vi "Manual Intake Mode.vi"(6 "Current Encoder Position":dbl) -> (1 "Rollers Active?":bool, 2 "Arm Power":dbl, 3 "Intake Power":dbl)   [LabVIEW 2015]
uses:
  Robot Global Data.vi
  <vilib>/addons/control/pid/pid.llb/PID (DBL).vi
  <vilib>/addons/control/pid/NI_PID_pid.lvlib
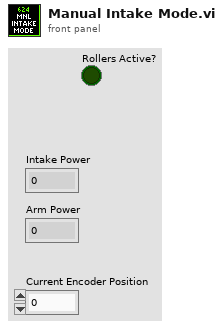
[diagram p1: front panel]
types:
  T1 = typedef "Dashboard Control Data.ctl" = cluster{"Encoder Control":T2, "Steer PID output":cluster{"output high":dbl, "output low":dbl}, " Steer PID gains":cluster{"proportional gain (Kc)":dbl, "integral time (Ti, min)":dbl, "derivative time (Td, min)":dbl}, "Drivetrain Settings":T3, "Vision Packet":T4, "Dashboard Drivetrain Command":T5, "Info/Command Cluster":T7, "Ball Vision Packet":T8, "Intake Presets":T10, "Intake Encoder Control":T12, "Climb Presets":T13, "Goal Output Range":cluster{"output high":dbl, "output low":dbl}, "Enabled Systems":T14, "Auton Presets":T15, "Pressure M":dbl, "Pressure B":dbl, "Vision Timeout":dbl, "Auto-Shift":T16, "Catapult Setpoints":T17}
  T2 = typedef "Encoder Control.ctl" = cluster{"Right Tick Constant":dbl, "Left Tick Constant":dbl, "Reset?":bool, "Y Dist":cluster{"PID gains":cluster{"proportional gain (Kc)":dbl, "integral time (Ti, min)":dbl, "derivative time (Td, min)":dbl}}, "Y Stop Thresh":dbl, "Y Stop Speed":dbl}
  T3 = typedef "Drivetrain Settings.ctl" = cluster{"Gyro Tolerance":dbl, "Throttle Ramp (ms)":dbl, "Kv":dbl, "Ka":dbl, "Feed Forward P":dbl, "Feed Forward D":dbl, "Goal Vision PID gains":cluster{"proportional gain (Kc)":dbl, "integral time (Ti, min)":dbl, "derivative time (Td, min)":dbl}, "Goal Detection Window":dbl, "Creep Rate":dbl, "Vision Throttle Threshold":dbl, "Min Turn Output":dbl, "Left Batter Angle":dbl, "Right Batter Angle":dbl}
  T4 = typedef "Goal Vision Packet.ctl" = cluster{"Distance":dbl, "Center X":dbl, "Center Y":dbl, "Found Target?":bool, "Robot Center":dbl, "Angle":dbl}
  T5 = typedef "Dashboard Drivetrain Command.ctl" = cluster{"Drivetrain Vision":T6}
  T6 = typedef "Drivetrain Vision.ctl" = cluster{"Goal Window":dbl, "Ball Window":dbl}
  T7 = typedef "Ball Tracking Command Cluster.ctl" = cluster{"Distance to Ball":dbl, "Desired Angle":dbl, "Command":enum16{"Turn to Ball", "Turn to Angle", "Get Distance"}, "Pixels from Center":dbl}
  T8 = typedef "Ball Vision Packet.ctl" = cluster{"Ball Detected?":bool, "Distance to Ball":dbl, "Desired Angle":dbl, "Pixels from Center":dbl, "Tracking mode":T9}
  T9 = typedef "Tracking Mode.ctl" = enum16{"Turn to Ball", "Turn to Angle"}
  T10 = typedef "Intake Presets.ctl" = cluster{"Intake Speed":dbl, "Outake Speed":dbl, "Angle Speed":dbl, "Angle Tolerance":dbl, "Encoder Scale":dbl, "Load Height":dbl, "Output Range":T11, "MaxCurrent":dbl, "Idle Height":dbl, "Max Height":dbl, "Reset Encoders?":bool, "PID gains":cluster{"proportional gain (Kc)":dbl, "integral time (Ti, min)":dbl, "derivative time (Td, min)":dbl}, "Drop Low Height ":dbl, "Rotation Power Max/Min":dbl}
  T11 = typedef "Drivetrain Output Range.ctl" = cluster{"output high":dbl, "output low":dbl}
  T12 = typedef "IntakeEcoderControl.ctl" = cluster{"Arm Tick Constant":dbl, "Reset?":bool, "Y Dist":cluster{"PID gains":cluster{"proportional gain (Kc)":dbl, "integral time (Ti, min)":dbl, "derivative time (Td, min)":dbl}}, "Y Stop Thresh":dbl, "Y Stop Speed":dbl}
  T13 = typedef "Climb Presets.ctl" = cluster{"Pull Power":dbl, "Extend Power":dbl}
  T14 = typedef "Enabled Systems.ctl" = cluster{"Shoot":bool, "Intake":bool, "DT":bool, "Gyro":bool, "100ms":bool, "US":bool}
  T15 = typedef "Autonomous Presets.ctl" = cluster{"Pitch Limit":dbl, "Roll Limit":dbl, "Start Position":dbl, "Cross Position":dbl}
  T16 = typedef "Auto Shift Cluster.ctl" = cluster{"Delay":dbl, "Speed Thresh":dbl, "Upshift Accel":dbl, "Upshift Throttle":dbl, "Upshift Throttle Accel":dbl, "Downshift Throttle":dbl, "Downshift Throttle Accel":dbl, "Pressure Threshold":dbl}
  T17 = typedef "Catapult Presets.ctl" = cluster{"Intake Danger Height":dbl, "Ball Security Delay ":dbl, "High PSI Minimum":dbl, "Shot Finish Delay":dbl, "Low PSI Minimum":dbl, "Idle Ball Security Wait ":dbl}
  T18 = typedef "Manual Intake Commands.ctl" = cluster{"Intake":bool, "Eject":bool, "Arm Angle":dbl, "Intake Override Speed":dbl, "Arm Override Speed":dbl, "Arm Speed":dbl, "Override Intake":bool, "Override Eject":bool, "Eject Override Speed":dbl, "Arm":bool, "Override Arm":bool, "Override Angle":bool}
  T19 = cluster{"proportional gain (Kc)":dbl, "integral time (Ti, min)":dbl, "derivative time (Td, min)":dbl}
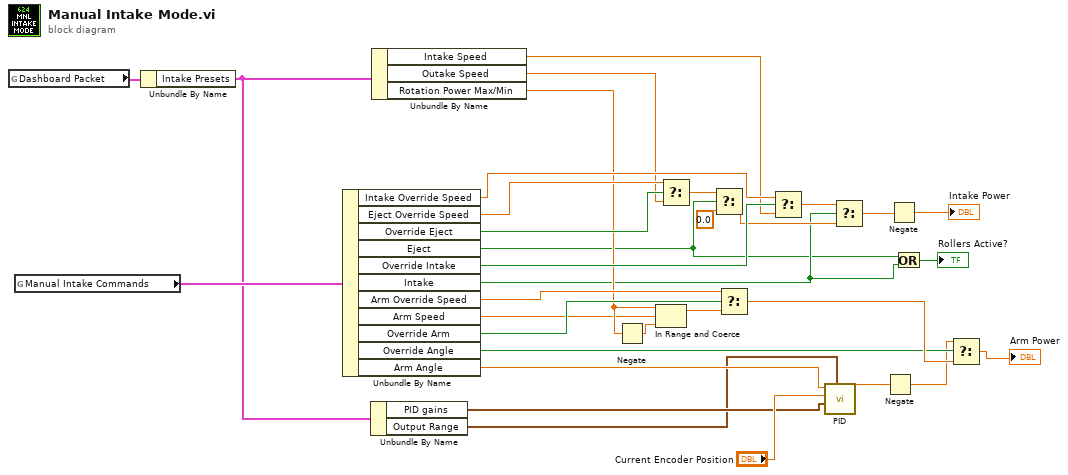
[diagram p0: block diagram]
diagram:
  n1 = global read "Robot Global Data.vi" "Dashboard Packet"() -> (w24:T1)
  n2 = global read "Robot Global Data.vi" "Manual Intake Commands"() -> (w21:T18)
  n3 = Unbundle By Name(w24) -> ("Intake Presets"=w8:T10)
  n4 = Unbundle By Name(w21) -> ("Intake Override Speed"=w27:dbl, "Eject Override Speed"=w33:dbl, "Override Eject"=w32:bool, "Eject"=w12:bool, "Override Intake"=w29:bool, "Intake"=w13:bool, "Arm Override Speed"=w25:dbl, "Arm Speed"=w17:dbl, "Override Arm"=w20:bool, "Override Angle"=w4:bool, "Arm Angle"=w10:dbl)
  n5 = Unbundle By Name(w8) -> ("PID gains"=w7:T19, "Output Range"=w6:T11)
  n6 = Unbundle By Name(w8) -> ("Intake Speed"=w23:dbl, "Outake Speed"=w22:dbl, "Rotation Power Max/Min"=w19:dbl)
  n7 = Negate(x=w19) -> (-x=w18:dbl)
  n8 = In Range and Coerce(upper limit=w19, x=w17, lower limit=w18) -> (coerced(x)=w16:dbl)  [unwired: 1 out]
  n9 = Select(t=w33, s=w32, f=w22) -> (s? t:f=w31:dbl)
  n10 = Select(t=w31, s=w12, f=0.0) -> (s? t:f=w26:dbl)
  n11 = Select(t=w25, s=w20, f=w16) -> (s? t:f=w5:dbl)
  n12 = Select(t=w27, s=w29, f=w23) -> (s? t:f=w30:dbl)
  n13 = call-poly <vilib>:"PID.vi"("output range"=w6, "PID gains"=w7, "process variable"="Current Encoder Position", "setpoint"=w10) -> ("output"=w3:dbl)  [unwired: 6 in, 1 out]
  n14 = Select(t=w30, s=w13, f=w26) -> (s? t:f=w15:dbl)
  n15 = Negate(x=w3) -> (-x=w2:dbl)
  n16 = Negate(x=w15) -> (-x=→"Intake Power":dbl)
  n17 = Or(x=w12, y=w13) -> (x .or. y?=→"Rollers Active?":bool)
  n18 = Select(t=w2, s=w4, f=w5) -> (s? t:f=→"Arm Power":dbl)
